vi "Single Channel Hex Gen.vi"(7 "System Clock(MHz)":dbl=240.0, 8 "RampOffset(ns)":i32, 9 "RampLength(ns)":i32=238310, 10 "Amplitude":dbl, 11 "Frequency":dbl) -> (2 "Single Freq Hex String":string)   [LabVIEW 2020]
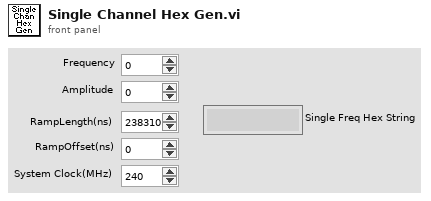
[diagram p1: front panel]
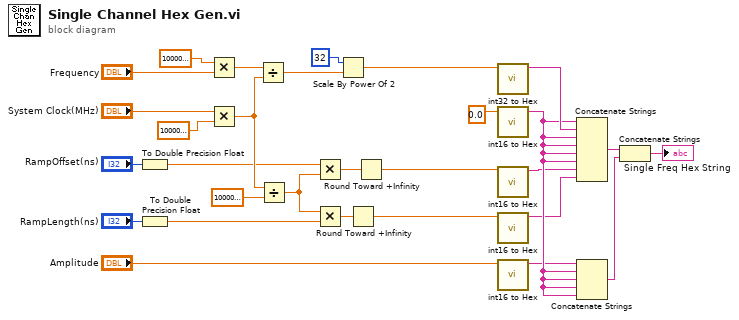
[diagram p0: block diagram]
diagram:
  n1 = To Double Precision Float(number="RampOffset(ns)") -> (double precision float=w17:dbl)
  n2 = To Double Precision Float(number="RampLength(ns)") -> (double precision float=w12:dbl)
  n3 = Multiply(x=1000000.0, y="Frequency") -> (x*y=w25:dbl)
  n4 = Multiply(x="System Clock(MHz)", y=1000000.0 ("x")) -> (x*y=w18:dbl)
  n5 = Divide(x=w25, y=w18) -> (x/y=w26:dbl)
  n6 = Divide(x=w18, y=1000000000.0) -> (x/y=w13:dbl)
  n7 = Multiply(x=w17, y=w13) -> (x*y=w21:dbl)
  n8 = Multiply(x=w13, y=w12) -> (x*y=w20:dbl)
  n9 = Scale By Power Of 2(n=32, x=w26) -> (x*2^n=w9:dbl)
  n10 = Round Toward +Infinity(x=w20) -> (ceil(x): smallest int >= x=w4:dbl)
  n11 = Round Toward +Infinity(x=w21) -> (ceil(x): smallest int >= x=w6:dbl)
  n12 = call "int32 to Hex.vi"("number"=w9) -> ("Hex string"=w10:string)  [unwired: 10 in]
  n13 = call "int16 to Hex.vi"("number"=0.0) -> ("Hex string"=w7:string)  [unwired: 10 in]
  n14 = call "int16 to Hex.vi"("number"=w6) -> ("Hex string"=w5:string)  [unwired: 10 in]
  n15 = call "int16 to Hex.vi"("number"=w4) -> ("Hex string"=w3:string)  [unwired: 10 in]
  n16 = call "int16 to Hex.vi"("number"="Amplitude") -> ("Hex string"=w2:string)  [unwired: 10 in]
  n17 = Concatenate Strings(w7, w10, w7, w7, w7, w7, w5, w3) -> (w29:string)
  n18 = Concatenate Strings(w2, w7, w7, w7, w7) -> (w28:string)
  n19 = Concatenate Strings(w29, w28) -> (→"Single Freq Hex String":string)
